vi "mainTest.vi"   [LabVIEW 2019]
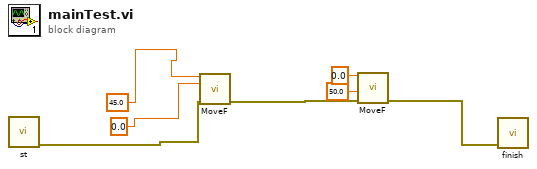
[diagram p0: block diagram]
diagram:
  n1 = call "st.vi"() -> ("Error/Flow Out"=w5:errorcluster)  [unwired: 11 in]
  n2 = call "MoveF.vi"("X"=45.0, "Y"=0.0, "error in (no error)"=w5) -> ("error out"=w4:errorcluster)  [unwired: 12 in]
  n3 = call "MoveF.vi"("X"=0.0, "Y"=50.0, "error in (no error)"=w4) -> ("error out"=w3:errorcluster)  [unwired: 12 in]
  n4 = call "finish.vi"("Error/Flow In"=w3) -> ()  [unwired: 11 in]
